vi "Polynomial Curve Fiting.vi"(3 "polynomial order":i32=2, 4 "end":dbl=1.0 format="%0.2f", 5 "start":dbl format="%0.2f", 6 "Y":dbl[](array[numeric]), 7 "X":dbl[](array[numeric])) -> (0 "T Last":dbl, 1 "T First":dbl, 2 "XY Graph":cluster{"Ramp Pattern":dbl[], dbl[]}(graph))   [LabVIEW 2017]
uses:
  <vilib>/Analysis/1siggen.llb/Ramp Pattern by Samples.vi
  <vilib>/Analysis/NI_AALBase.lvlib
  <vilib>/Analysis/NI_AALPro.lvlib
panel:
  out "XY Graph 2":cluster{"Ramp Pattern":dbl[], dbl[]}(graph)
  in  "samples":i32=128
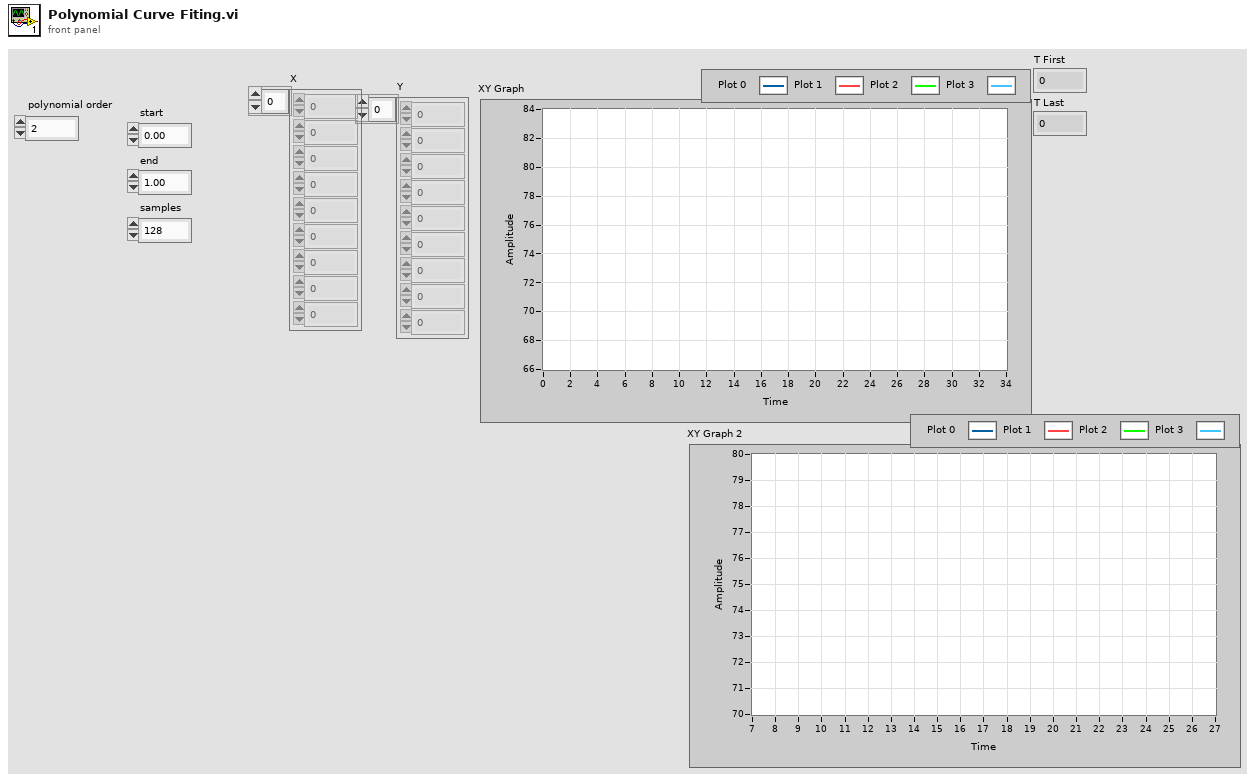
[diagram p1: front panel]
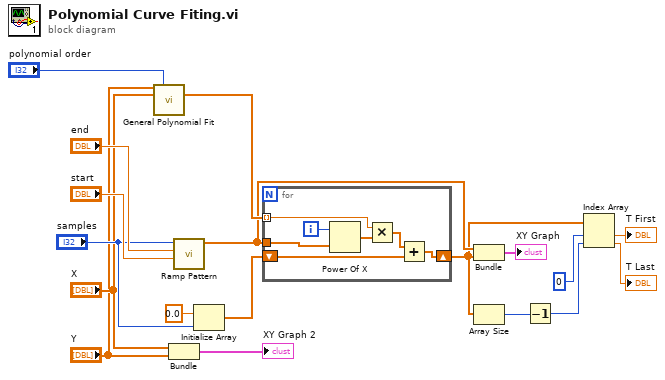
[diagram p0: block diagram]
diagram:
  n1 = call <vilib>:"General Polynomial Fit.vi"("Y"="Y", "polynomial order"="polynomial order", "X"="X") -> ("Polynomial Coefficients"=w18:dbl[])  [unwired: 9 in, 3 out]
  n2 = Bundle("X"="X", "Y"="Y") -> (→"XY Graph 2":cluster{"X":dbl[], "Y":dbl[]})  [unwired: 1 in]
  n3 = call-poly <vilib>:"Ramp Pattern.vi"("start"="start", "end"="end", "samples"="samples") -> ("Ramp Pattern"=w14:dbl[])  [unwired: 7 in, 1 out]
  n4 = Initialize Array(0.0 ("element"), "samples") -> (w15:dbl[])
  n5 = for {
    tunnel: w18 -> [w22] mode=indexing
    tunnel: w14 -> [w25]
    shift-right: [w20] -> w8
    shift-left: w15 -> [w19]
    i -> [w24]
    n6 = Power Of X(1:w25, 2:w24) -> (0:w23:dbl[])
    n7 = Multiply(x=w22, y=w23) -> (x*y=w21:dbl[])
    n8 = Add(x=w21, y=w19) -> (x+y=w20:dbl[])
  }
  n9 = Bundle("Ramp Pattern"=w14, w8) -> (→"XY Graph":cluster{"Ramp Pattern":dbl[], dbl[]})  [unwired: 1 in]
  n10 = Array Size(array=w8) -> (size(s)=w7:i32)
  n11 = Decrement(x=w7) -> (x-1=w6:i32)
  n12 = Index Array(array=w8, index #1=0 ("index"), index #2=w6) -> (element #1=→"T First":dbl, element #2=→"T Last":dbl)
